vi "PCert-Container-Construct.vi"(6 "FTW Actor Instance Configuration":string="{\n  \"Identity\": \"ActorName\",\n  \"InboxAddress\": \"tcp://127.0.0.1:*\",\n  \"PublisherAddress\": \"tcp://127.0.0.1:*\",\n  \"DebugEnableInboxLogging\": false,\n  \"DebugEnableJobLogging\": false,\n  \"DebugShowPanel\": false\n}", 8 "error in (no error)":errorcluster, 11 "Initialization Sequence":string="FTW: Initialize") -> (0 "error out":errorcluster, 3 "ERP-Container-UI out":refnum<class "PCert-Container-UI.lvclass">)   [LabVIEW 2013, in "PCert-Container-UI.lvclass"]
uses:
  PCert-Container-UI.lvclass
  PCert-Container-UI.lvclass/PCert-Container-UI.ctl
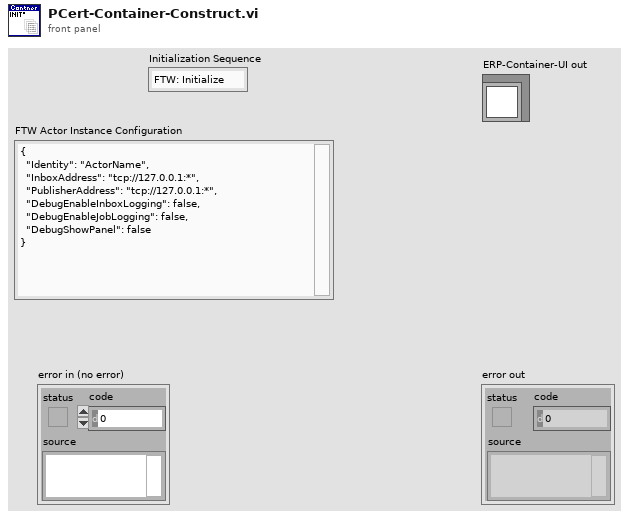
[diagram p1: front panel]
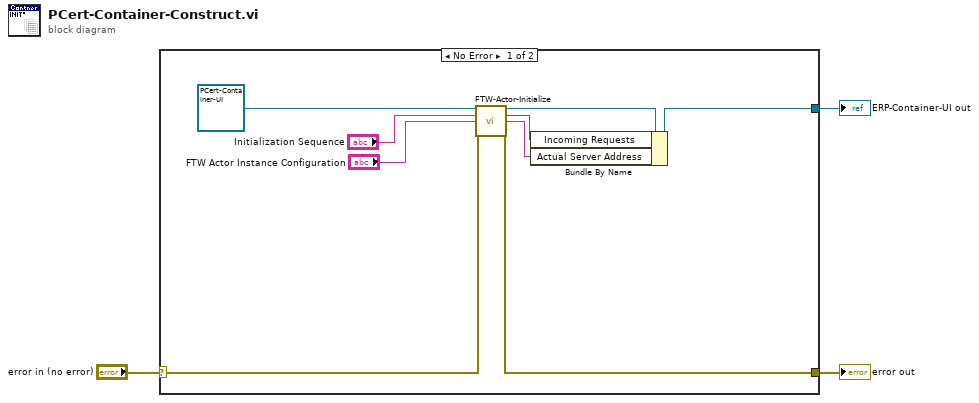
[diagram p0: block diagram]
diagram:
  n1 = case shown="No Error" "error in (no error)" {
    selector: "error in (no error)" -> [w10 w13]
    tunnel: [w7 w13] -> w2
    tunnel: [w4 _] -> w1
    frame No Error {
      n2 = call-dynamic "FTW-Actor-Initialize.vi"("FTW Actor Instance Type"=refnum<class "PCert-Container-UI.lvclass"> refnum ("ERP-Container-UI.lvclass"), "Initialization Job Sequence"="Initialization Sequence", "Actor Instance Configuration"="FTW Actor Instance Configuration", "error in"=w10) -> ("FTW Actor Instance"=w9:refnum<class "PCert-Container-UI.lvclass">, "Incoming Requests"=w8:refnum<event-registration>, "Actual Server Address"=w5:string, "error out"=w7:errorcluster)  [unwired: 8 in]
      n3 = Bundle By Name(cluster=w9, "Incoming Requests"=w8, "Actual Server Address"=w5) -> (w4:refnum<class "PCert-Container-UI.lvclass">)
    }
    frame Error {
    }
  }
  "error out" <- w2
  "ERP-Container-UI out" <- w1
